vi "Lidar Chirp Global.vi"() -> ()   [LabVIEW 2009]
panel:
  in  "Cluster":cluster{}
  out "Lidar Chirp Frequency, in pi rad (?Hz)(100KHz)":fxp<+/-,20,1>
  out "Lidar Mass Cancelling Gain":fxp<+/-,10,1>
  out "Lidar Phi_ M":fxp<+/-,10,1>
  out "Lidar Phi_Lidar - Phi_A":fxp<+/-,10,1>
  out "Lidar Phi_Lidar":fxp<+/-,10,1>
  out "Lidar Phi_B":fxp<+/-,10,1>
  out "Lidar Phi_A":fxp<+/-,10,1>
  out "Lidar Speed, Measured (ft/sec)":fxp<+/-,14,4>
  out "Lidar Speed Control Integral Feedback Gain":fxp<+/-,20,5>
  out "Lidar Speed Control Feedback Gain":fxp<+/-,20,5>
  out "Lidar Phi_B Set Point (pi rad)":fxp<+/-,14,4>
  out "Mechanical Advantage phi_a/phi_b":fxp<+/-,8,1>
  out "Voltage Amplitude":fxp<+/-,20,5>
  out "Output Voltage":fxp<+/-,20,5>
  # "X must be zero for this code to work.\nOtherwise I would have to redo the\nlookup tables for the new X"
  # "Phi_B is the Motor Crank\nPhi_A is the Rocker\n\nBoth are in units of pi radians"
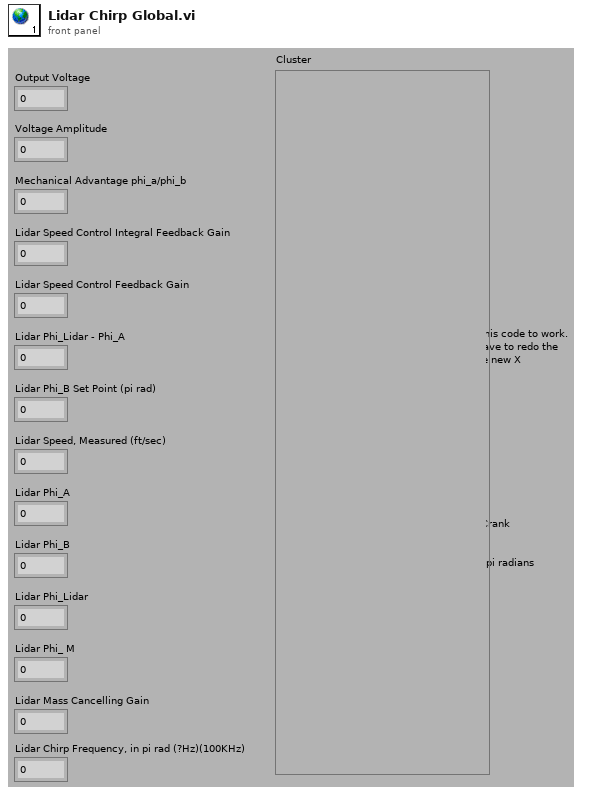
[diagram p1: front panel]
diagram:
